vi "Stop Core.vi"(10 "final error code":i32, 11 "CS++SVMonitor in":refnum<class "CS++SVMonitor.lvclass">) -> (3 "CS++SVMonitor out":refnum<class "CS++SVMonitor.lvclass">)   [LabVIEW 2012, in "CS++SVMonitor.lvlib" / "CS++SVMonitor.lvclass"]
doc: "(<B>Filename</B>: Actor Framework.lvlib:Actor.lvclass:Stop Core.vi)\n\nDefines what the actor does before it stops. Use the <B>final error code</B> input to determine whether the actor shut down in response to an error.\n\nBy default, this method does nothing. A descendant class may override it to define behavior, such as shutting down any processes the actor initiated in its override of the Actor Core method."
uses:
  CS++SVMonitor.lvclass
  CS++PVMonitor/CS++PVMonitor.lvclass
  CS++SVMonitor.lvclass/CS++SVMonitor.ctl
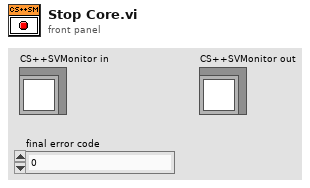
[diagram p1: front panel]
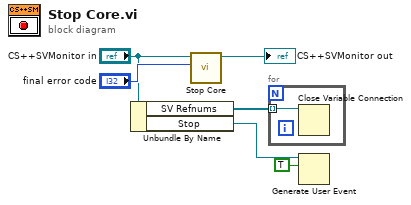
[diagram p0: block diagram]
diagram:
  n1 = Unbundle By Name("CS++SVMonitor in") -> ("SV Refnums"=w3:refnum<k21>[], "Stop"=w2:refnum<user-event>)
  n2 = call-parent "Stop Core.vi"("final error code"="final error code", "CS++BaseActor in"="CS++SVMonitor in") -> ("CS++BaseActor out"=→"CS++SVMonitor out":refnum<class "CS++SVMonitor.lvclass">)  [unwired: 9 in]
  n3 = for {
    tunnel: w3 -> [w7] mode=indexing
    n4 = Close Variable Connection(11:w7) -> ()  [unwired: 1 in, 1 out]
  }
  n5 = Generate User Event(user event=w2, event data cluster=TRUE ("event data")) -> ()  [unwired: 1 in, 2 out]
